vi "Laser_order_controller_vi.vi"(8 "error in":errorcluster, 11 "Laser Toggles":T1 {"Laser 488 order selection" items=["Not active", "1", "2", "3", "4"]; "Laser 642 order selection" items=["Not active", "1", "2", "3", "4"]; "Laser 595 order selection" items=["Not active", "1", "2", "3", "4"]; "Laser 560 order selection" items=["Not active", "1", "2", "3", "4"]; "Laser 642 nm power" min=0.0 max=5.0 scale=0.0..100.0; "Laser 595 nm power" min=0.0 max=5.0 scale=0.0..100.0; "Laser 560 nm power" min=0.0 max=5.0 scale=0.0..100.0; "Laser 488 nm power" min=0.0 max=5.0 scale=0.0..100.0}) -> (0 "error out":errorcluster, 1 "Active lasers":i16, 2 "Digital Waveform Graph":digitalwaveform(graph))   [LabVIEW 2020]
uses:
  Test project/typedefs/Laser_toggles_typedef.ctl
  <vilib>/Waveform/DWDTOps.llb/DWDT Compress Digital.vi
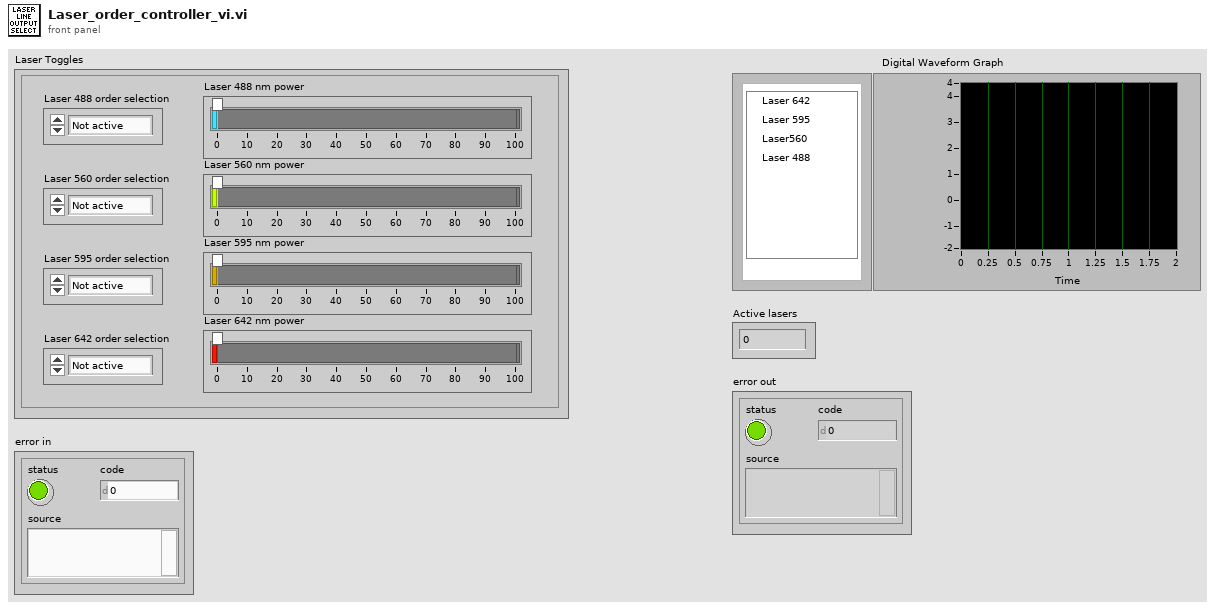
[diagram p1: front panel]
types:
  T1 = typedef "Laser_toggles_typedef.ctl" = cluster{"Laser 488 nm power":dbl, "Laser 560 nm power":dbl, "Laser 595 nm power":dbl, "Laser 642 nm power":dbl, "Laser 560 order selection":u16, "Laser 595 order selection":u16, "Laser 642 order selection":u16, "Laser 488 order selection":u16}
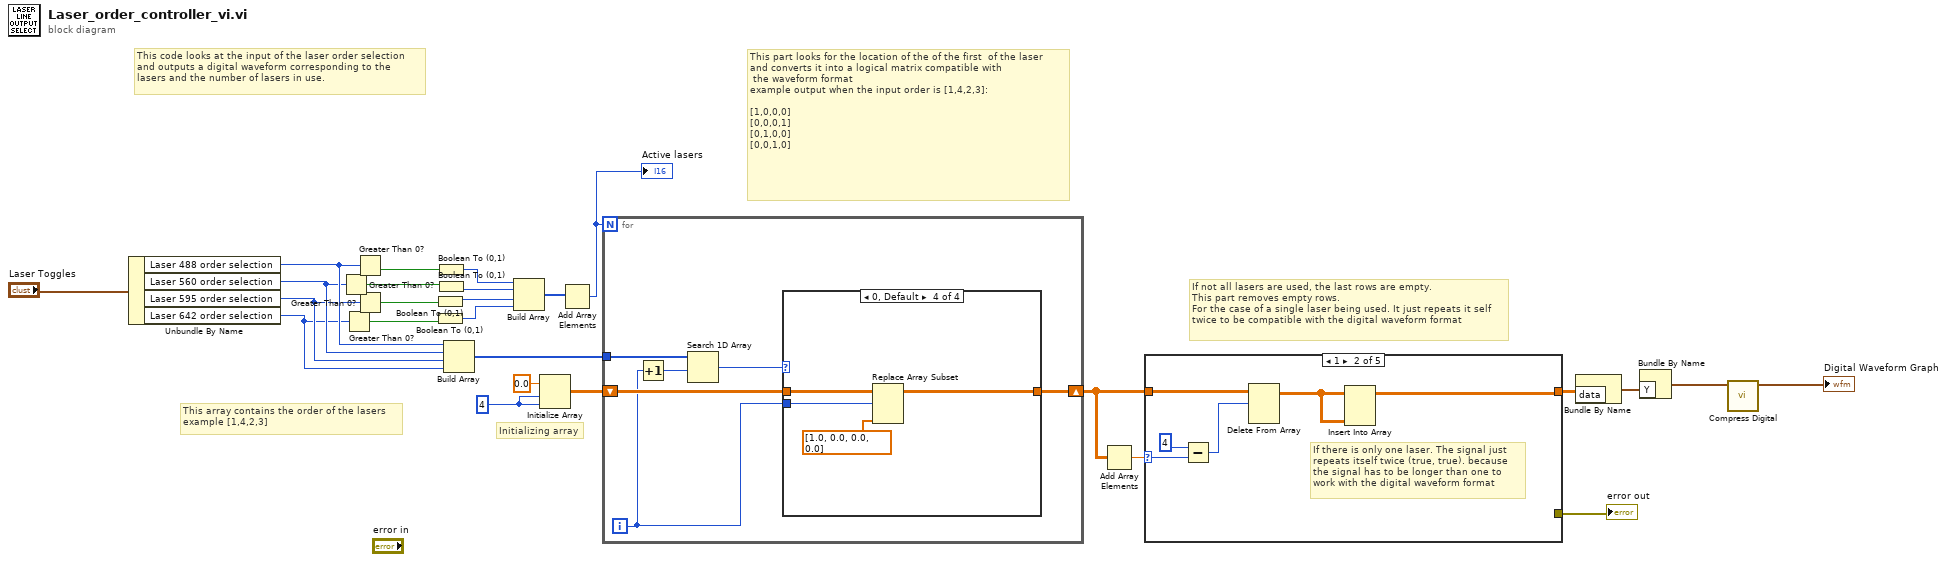
[diagram p0: block diagram]
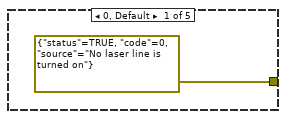
[diagram p2: hidden frame]
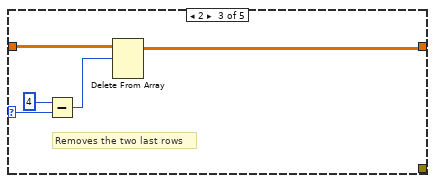
[diagram p3: hidden frame]
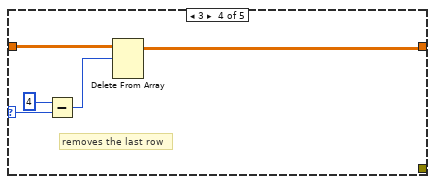
[diagram p4: hidden frame]
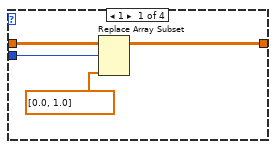
[diagram p6: hidden frame]
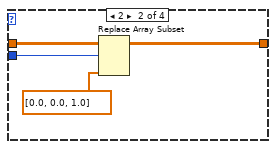
[diagram p7: hidden frame]
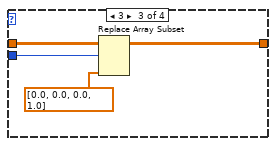
[diagram p8: hidden frame]
diagram:
  w17 = 4
  # "This code looks at the input of the laser order selection\nand outputs a digital waveform corresponding to the \nlasers and the number of lasers in use."
  # "If not all lasers are used, the last rows are empty.\nThis part removes empty rows.\nFor the case of a single laser being used. It just repeats it self\ntwice to be compatible with the digital waveform format"
  # "This array contains the order of the lasers \nexample [1,4,2,3]"
  # "This part looks for the location of the of the first  of the laser \nand converts it into a logical matrix compatible with\n the waveform format  \nexample output when the input order is [1,4,2,3]:\n\n[1,0,0,0]\n[0,0,0,1]\n[0,1,0,0]\n[0,0,1,0]"
  # "Initializing array"
  n1 = Unbundle By Name("Laser Toggles") -> ("Laser 488 order selection"=w7:u16, "Laser 560 order selection"=w6:u16, "Laser 595 order selection"=w5:u16, "Laser 642 order selection"=w4:u16)
  n2 = Greater Than 0?(x=w6) -> (x > 0?=w13:bool)
  n3 = Greater Than 0?(x=w4) -> (x > 0?=w11:bool)
  n4 = Greater Than 0?(x=w7) -> (x > 0?=w14:bool)
  n5 = Greater Than 0?(x=w5) -> (x > 0?=w12:bool)
  n6 = Boolean To (0,1)(Boolean=w12) -> (0, 1=w24:i16)
  n7 = Boolean To (0,1)(Boolean=w11) -> (0, 1=w23:i16)
  n8 = Boolean To (0,1)(Boolean=w14) -> (0, 1=w26:i16)
  n9 = Boolean To (0,1)(Boolean=w13) -> (0, 1=w25:i16)
  n10 = Build Array(w7, w6, w5, w4) -> (w19:u16[])
  n11 = Build Array(w26, w25, w24, w23) -> (w22:i16[])
  n12 = Initialize Array(0.0 ("element"), w17, w17) -> (w20:dbl[][])
  n13 = Add Array Elements(numeric array=w22) -> (sum=w3:i16)
  "Active lasers" <- w3
  n14 = for {
    N: w3 -> [_]
    tunnel: w19 -> [w32]
    shift-right: [w28] -> w15
    shift-left: w20 -> [w29]
    i -> [w27]
    n15 = Increment(x=w27) -> (x+1=w31:i32)
    n16 = Search 1D Array(1D array=w32, element=w31) -> (index of element=w30:i32)  [unwired: 1 in]
    n17 = case shown="0, Default" w30 {
      tunnel: w29 -> [w36 w40 w44 w48]
      tunnel: [w35 w39 w43 w47] -> w28
      tunnel: w27 -> [w34 w38 w42 w45]
      frame 1 {
        n18 = Replace Array Subset(array=w36, new element=dbl[] [0.0, 1.0] ("new element/subarray"), index (row)=w34) -> (w35:dbl[][])  [unwired: 1 in]
      }
      frame 2 {
        n19 = Replace Array Subset(array=w40, new element=dbl[] [0.0, 0.0, 1.0] ("new element/subarray"), index (row)=w38) -> (w39:dbl[][])  [unwired: 1 in]
      }
      frame 3 {
        n20 = Replace Array Subset(array=w44, new element=dbl[] [0.0, 0.0, 0.0, 1.0] ("new element/subarray"), index (row)=w42) -> (w43:dbl[][])  [unwired: 1 in]
      }
      frame 0, Default {
        n21 = Replace Array Subset(array=w48, new element=dbl[] [1.0, 0.0, 0.0, 0.0] ("new element/subarray"), index (row)=w45) -> (w47:dbl[][])  [unwired: 1 in]
      }
    }
  }
  n22 = Add Array Elements(numeric array=w15) -> (sum=w16:dbl)
  n23 = case shown="1" w16 {
    selector: w16 -> [_ w53 w58 w63 _]
    tunnel: w15 -> [_ w55 w60 w65 w66]
    tunnel: [_ w50 w56 w61 w66] -> w10
    tunnel: [errorcluster {"status"=TRUE, "code"=0, "source"="No laser line is turned on"} ("error constant") _ _ _ _] -> w2
    frame 0, Default {
    }
    frame 1 {
      # "If there is only one laser. The signal just repeats itself twice (true, true). because the signal has to be longer than one to work with the digital waveform format"
      n24 = Subtract(x=4, y=w53) -> (x-y=w52:i32)
      n25 = Delete From Array(array=w55, length=w52) -> (array with subset deleted=w51:dbl[][])  [unwired: 2 in, 1 out]
      n26 = Insert Into Array(array=w51, new element=w51) -> (w50:dbl[][])  [unwired: 2 in]
    }
    frame 2 {
      # "Removes the two last rows"
      n27 = Subtract(x=4, y=w58) -> (x-y=w57:i32)
      n28 = Delete From Array(array=w60, length=w57) -> (array with subset deleted=w56:dbl[][])  [unwired: 2 in, 1 out]
    }
    frame 3 {
      # "removes the last row"
      n29 = Subtract(x=4, y=w63) -> (x-y=w62:i32)
      n30 = Delete From Array(array=w65, length=w62) -> (array with subset deleted=w61:dbl[][])  [unwired: 2 in, 1 out]
    }
    frame 4 {
    }
  }
  "error out" <- w2
  n31 = Bundle By Name("data"=w10) -> (w18:digitaldata)  [unwired: 1 in]
  n32 = Bundle By Name("Y"=w18) -> (w9:digitalwaveform)  [unwired: 1 in]
  n33 = call-poly <vilib>:"Compress Digital.vi"("uncompressed digital waveform"=w9) -> ("compressed digital waveform"=→"Digital Waveform Graph":digitalwaveform)  [unwired: 9 in, 1 out]
